vi "process.vi"(8 "error in (no error)":errorcluster, 11 "Project in":refnum<class "Project.lvclass">) -> (0 "error out":errorcluster, 3 "Project out":refnum<class "Project.lvclass">)   [LabVIEW 2016, in "Project.lvclass"]
uses:
  Project.lvclass
  Search/Search.lvclass
  Project.lvclass/Project.ctl
  Search/Search.lvclass/Search.ctl
  ProjectItem/ProjectItem.lvclass/ProjectItem.ctl
  IProjectItemFactory/IProjectItemFactory.lvclass
  ProjectItem/ProjectItem.lvclass
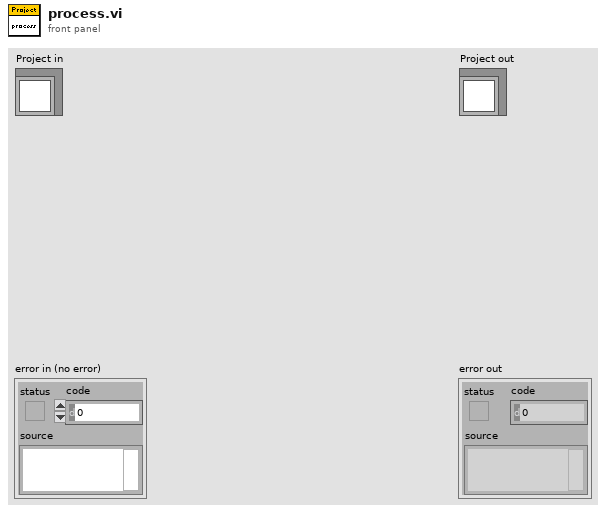
[diagram p1: front panel]
types:
  T1 = cluster{"OldLibrary":string, "NewLibrary":string}
  T2 = typedef "LibraryDirectories.ctl" = cluster{"OldLibraryDirectory":string, "NewLibraryDirectory":string}
  T3 = typedef "LibraryMemberNameReplacement.ctl" = cluster{"String To Replace in VI names":string, "String To Replace in Control names":string, "New String in VI names":string, "New String in Control names":string}
  T4 = typedef "ProjectItemSelection.ctl" = enum16{"Default", "ClassPrivateData", "Dependencies", "Folder", "Library", "LVClass", "VI"}
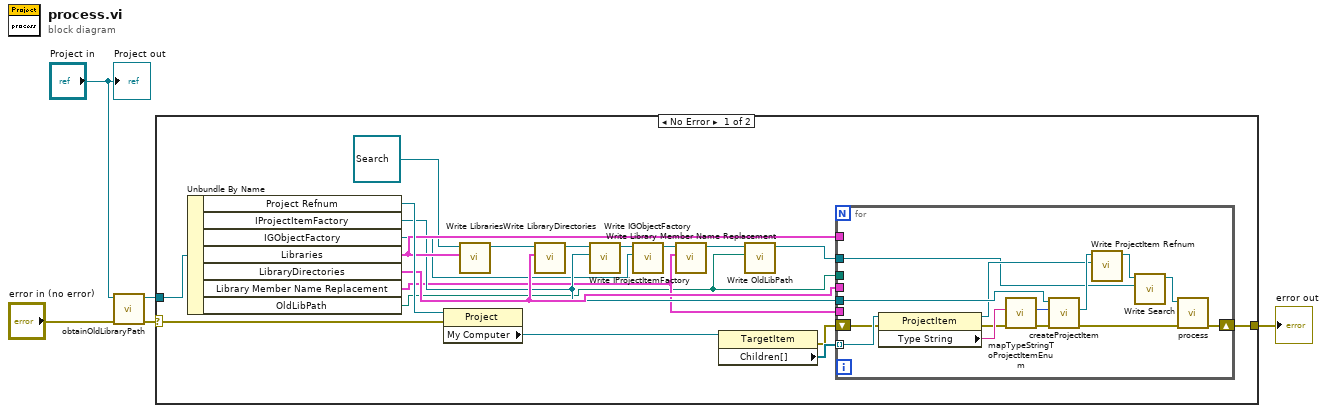
[diagram p0: block diagram]
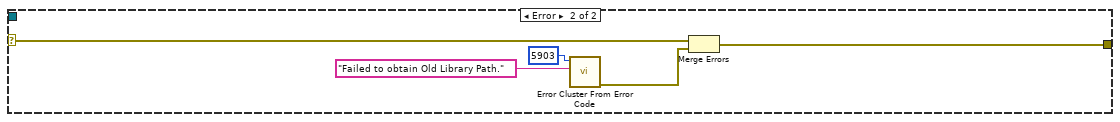
[diagram p2: hidden frame]
diagram:
  n1 = call "obtainOldLibraryPath.vi"("error in (no error)"="error in (no error)", "Project in"="Project in") -> ("error out"=w3:errorcluster, "Project out"=w4:refnum<class "Project.lvclass">)  [unwired: 7 in, 1 out]
  n2 = case shown="No Error" w3 {
    selector: w3 -> [w20 w44]
    tunnel: w4 -> [w22 _]
    tunnel: [w21 w40] -> w1
    frame No Error {
      n3 = Unbundle By Name(w22) -> ("Project Refnum"=w24:refnum<vi>, "IProjectItemFactory"=w12:refnum<class "IProjectItemFactory.lvclass">, "IGObjectFactory"=w7:refnum<class "IGObjectFactory.lvclass">, "Libraries"=w18:T1, "LibraryDirectories"=w13:T2, "Library Member Name Replacement"=w11:T3, "OldLibPath"=w10:path)
      n4 = property class="Project"(reference=w24, error in=w20) -> ("My Computer"=w25:refnum<vi>)  [unwired: 2 out]
      n5 = call "Write Libraries.vi"("Libraries"=w18, "ProjectItem in"=refnum<class "Search.lvclass"> refnum ("Search.lvclass")) -> ("ProjectItem out"=w16:refnum<class "Search.lvclass">)  [unwired: 9 in]
      n6 = call "Write LibraryDirectories.vi"("LibraryDirectories"=w13, "ProjectItem in"=w16) -> ("ProjectItem out"=w15:refnum<class "Search.lvclass">)  [unwired: 9 in]
      n7 = call "Write IProjectItemFactory.vi"("IProjectItemFactory"=w12, "ProjectItem in"=w15) -> ("ProjectItem out"=w6:refnum<class "Search.lvclass">)  [unwired: 9 in]
      n8 = call "Write IGObjectFactory.vi"("IGObjectFactory"=w7, "Search in"=w6) -> ("Search out"=w8:refnum<class "Search.lvclass">)  [unwired: 9 in]
      n9 = call "Write Library Member Name Replacement.vi"("Library Member Name Replacement"=w11, "ProjectItem in"=w8) -> ("ProjectItem out"=w14:refnum<class "Search.lvclass">)  [unwired: 9 in]
      n10 = property class="TargetItem"(reference=w25) -> (error out=w19:errorcluster, "Children[]"=w23:refnum<vi>[])  [unwired: 1 in, 1 out]
      n11 = call "Write OldLibPath.vi"("OldLibPath"=w10, "ProjectItem in"=w14) -> ("ProjectItem out"=w9:refnum<class "Search.lvclass">)  [unwired: 9 in]
      n12 = for {
        tunnel: w23 -> [w39] mode=indexing
        tunnel: w12 -> [w35]
        tunnel: w18 -> [_]
        tunnel: w11 -> [_]
        tunnel: w10 -> [_]
        tunnel: w13 -> [_]
        shift-right: [w31] -> w21
        shift-left: w19 -> [w30]
        tunnel: w9 -> [w26]
        n13 = property class="ProjectItem"(reference=w39, error in=w30) -> (reference out=w34:refnum<vi>, error out=w29:errorcluster, "Type String"=w38:string)
        n14 = call "mapTypeStringToProjectItemEnum.vi"("error in (no error)"=w29, "Type String"=w38) -> ("error out"=w33:errorcluster, "ProjectItemSelection"=w37:T4)  [unwired: 7 in, 1 out]
        n15 = call-dynamic "createProjectItem.vi"("error in (no error)"=w33, "ProjectItemSelection"=w37, "IProjectItemFactory in"=w35) -> ("error out"=w32:errorcluster, "ProjectItem"=w36:refnum<class "ProjectItem.lvclass">)  [unwired: 6 in, 1 out]
        n16 = call "Write ProjectItem Refnum.vi"("ProjectItem Refnum"=w34, "ProjectItem in"=w36) -> ("ProjectItem out"=w28:refnum<class "ProjectItem.lvclass">)  [unwired: 9 in]
        n17 = call "Write Search.vi"("Search"=w26, "ProjectItem in"=w28) -> ("ProjectItem out"=w27:refnum<class "ProjectItem.lvclass">)  [unwired: 9 in]
        n18 = call-dynamic "process.vi"("error in (no error)"=w32, "ProjectItem in"=w27) -> ("error out"=w31:errorcluster)  [unwired: 8 in, 1 out]
      }
    }
    frame Error {
      n19 = call <vilib>:"Error Cluster From Error Code.vi"("error message (\"\")"="Failed to obtain Old Library Path." ("error message (\"\")"), "error code (0)"=5903) -> ("error out"=w41:errorcluster)  [unwired: 7 in]
      n20 = Merge Errors(w44, w41) -> (w40:errorcluster)
    }
  }
  "error out" <- w1
  "Project out" <- "Project in"
